vi "Start.vi"(8 "error in (no error)":errorcluster, 11 "Electrophysiology in":refnum<class "IntanElectrophysiology.lvclass">) -> (0 "error out":errorcluster, 3 "Electrophysiology out":refnum<class "IntanElectrophysiology.lvclass">)   [LabVIEW 2014, in "IntanElectrophysiology.lvclass"]
uses:
  IntanElectrophysiology.lvclass
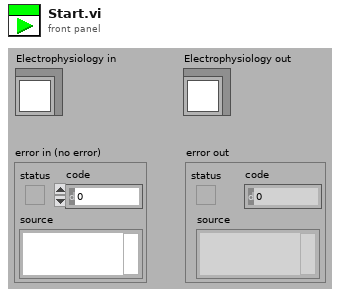
[diagram p1: front panel]
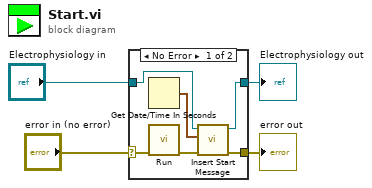
[diagram p0: block diagram]
diagram:
  n1 = case shown="No Error" "error in (no error)" {
    selector: "error in (no error)" -> [w5 w12]
    tunnel: [w6 w12] -> w4
    tunnel: [w9 w11] -> w1
    tunnel: "Electrophysiology in" -> [w7 w11]
    frame No Error {
      n2 = Get Date/Time In Seconds() -> (seconds since 1Jan1904=w10:timestamp)
      n3 = call "Run.vi"("error in (no error)"=w5) -> ("error out"=w8:errorcluster)  [unwired: 9 in, 1 out]
      n4 = call-dynamic "Insert Start Message.vi"("error in (no error)"=w8, "Start Time"=w10, "Electrophysiology in"=w7) -> ("error out"=w6:errorcluster, "Electrophysiology out"=w9:refnum<class "IntanElectrophysiology.lvclass">)  [unwired: 7 in]
    }
    frame Error {
    }
  }
  "error out" <- w4
  "Electrophysiology out" <- w1
